vi "XY Graph TipStrip Mouse Move.vi"(4 "Top/Bottom(F)":bool, 5 "Max Length (200)":i32=200, 6 "Left/Right(F)":bool, 7 "Offset (10)":i32=10, 8 "Error In":errorcluster, 10 "Coords":T1, 11 "XY Graph Refnum":T2) -> (0 "Error Out":errorcluster, 1 "Plot Name":string, 2 "Plot at Coordinates":i32)   [LabVIEW 2019, in "XY Graph Add-Ons.lvlib"]
doc: "Shows a tipstrip indicating the name of the plot in the graph legend over which the mouse is located.\n\nThe maximal length (<b>Max Length</b>)of the tipstrip is optional (default: 200 pixels).\nThe relative location of the tipstrip (with respect to the mouse) can be specified with two flags (<b>Top/Bottom</b> and <b>Left/Right</b>) and an <b>Offset</b> value.\nThe default is bottom right, with an offset of 10 pixels in both directions.\n\nIf the mouse is over a plot legend, its index and legend are returned. Otherwise -1 and an empty string are returned."
uses:
  XY Graph Add-Ons.lvlib
  XY Graph Refnum.ctl
  <vilib>/Utility/miscctls.llb/LVPoint32TypeDef.ctl
  <vilib>/Utility/miscctls.llb/LVPositionTypeDef.ctl
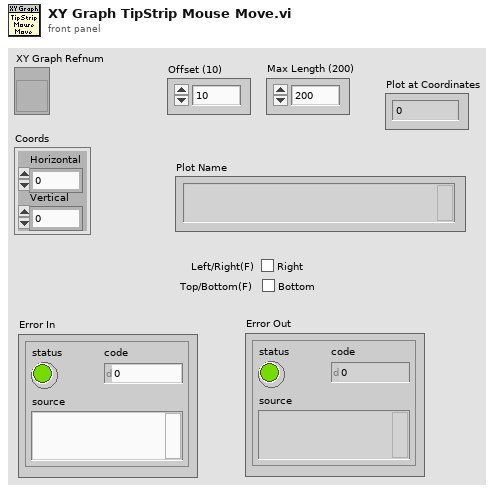
[diagram p1: front panel]
types:
  T1 = typedef "LVPoint32TypeDef.ctl" = cluster{"Horizontal":i32, "Vertical":i32}
  T2 = typedef "XY Graph Add-Ons.lvlib/XY Graph Refnum.ctl" = refnum<vi>
  T3 = typedef "LVPositionTypeDef.ctl" = cluster{"Left":i32, "Top":i32}
  T4 = typedef "LVPointTypeDef.ctl" = cluster{"Horizontal":i16, "Vertical":i16}
  T5 = typedef "LVBoundsTypeDef.ctl" = cluster{"Width":u32, "Height":u32}
  T6 = cluster{"left":i16, "top":i16, "right":i16, "bottom":i16}
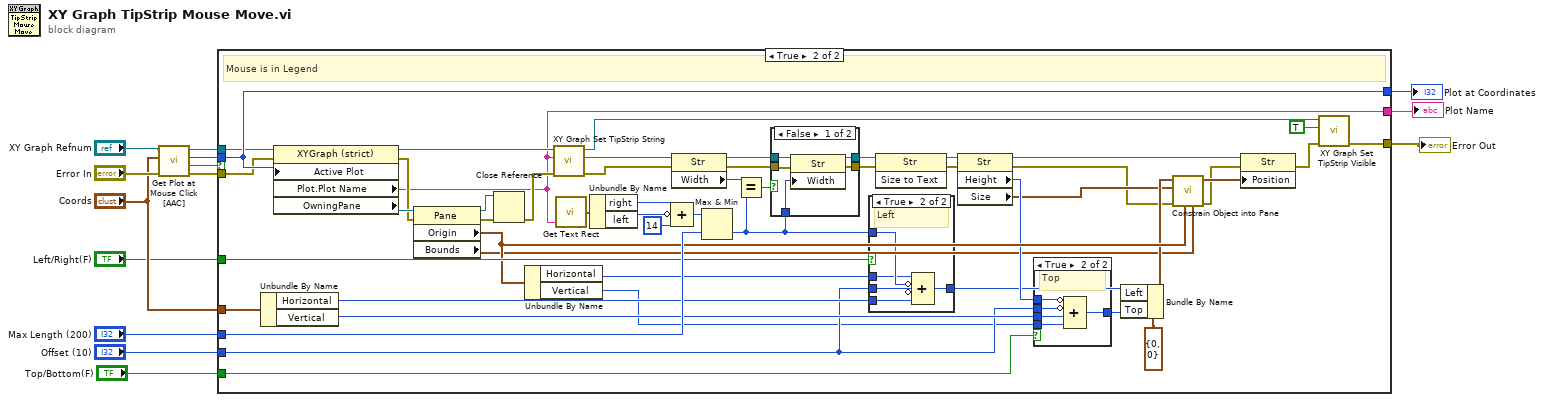
[diagram p0: block diagram]
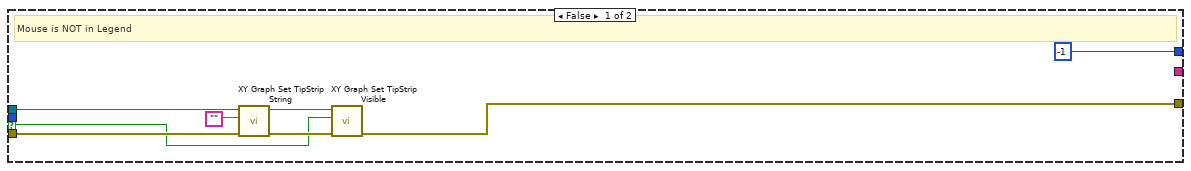
[diagram p2: hidden frame]
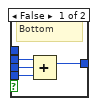
[diagram p3: hidden frame]
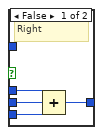
[diagram p4: hidden frame]
diagram:
  n1 = call "Get Plot at Mouse Click [AAC].vi"("error in (no error)"="Error In", "Mouse Click Coordinates"="Coords", "XYGraph Ref"="XY Graph Refnum") -> ("error out"=w1:errorcluster, "Click is in Legend?"=w12:bool, "Plot at Coordinates"=w11:i32, "XYGraph Ref"=w2:T2)  [unwired: 2 in, 3 out]
  n2 = case shown="True" w12 {
    selector: w12 -> [w18 _]
    tunnel: w11 -> [_ w63]
    tunnel: [w16 w26] -> w10
    tunnel: "Coords" -> [_ w71]
    tunnel: [_ w24] -> w8
    tunnel: "Max Length (200)" -> [_ w73]
    tunnel: "Left/Right(F)" -> [_ w72]
    tunnel: "Top/Bottom(F)" -> [_ w70]
    tunnel: "Offset (10)" -> [_ w67]
    tunnel: [-1 ("Plot at Coordinates") w63] -> w3
    tunnel: w2 -> [w17 w60]
    tunnel: w1 -> [w20 w33]
    frame False {
      # "Mouse is NOT in Legend"
      n3 = call "XY Graph Set TipStrip String.vi"("error in (no error)"=w20, "TipStrip String"="", "XY Graph Refnum"=w17) -> ("error out"=w19:errorcluster, "XY Graph Refnum (dup)"=w15:T2)  [unwired: 6 in, 1 out]
      n4 = call "XY Graph Set TipStrip Visible.vi"("error in (no error)"=w19, "TipStrip Visible"=w18, "XY Graph Refnum"=w15) -> ("error out"=w16:errorcluster)  [unwired: 6 in, 2 out]
    }
    frame True {
      # "Mouse is in Legend"
      n5 = Unbundle By Name(w71) -> ("Horizontal"=w68:i32, "Vertical"=w69:i32)
      n6 = property class="XYGraph (strict)"(reference=w60, error in=w33, "Active Plot"=w63) -> (reference out=w32:T2, error out=w65:errorcluster, "Plot.Plot Name"=w24:string, "OwningPane"=w66:refnum<vi>)
      n7 = property class="Pane"(reference=w66, error in=w65) -> (reference out=w62:refnum<vi>, error out=w61:errorcluster, "Origin"=w64:T4, "Bounds"=w23:T5)
      n8 = Close Reference(reference=w62, error in (no error)=w61) -> (error out=w29:errorcluster)
      n9 = Unbundle By Name(w64) -> ("Horizontal"=w37:i16, "Vertical"=w36:i16)
      n10 = call "XY Graph Set TipStrip String.vi"("error in (no error)"=w29, "TipStrip String"=w24, "XY Graph Refnum"=w32) -> ("error out"=w30:errorcluster, "TipStrip Refnum"=w31:refnum<vi>, "XY Graph Refnum (dup)"=w28:T2)  [unwired: 6 in]
      n11 = call <vilib>:"Get Text Rect.vi"("text"=w24) -> ("rect"=w59:T6)  [unwired: 8 in]
      n12 = Unbundle By Name(w59) -> ("right"=w58:i16, "left"=w57:i16)
      n13 = Compound Arithmetic op=ADD(w58, invert w57, i16 14 ("value")) -> (w55:i16)
      n14 = property class="Str"(reference=w31, error in=w30) -> (reference out=w52:refnum<vi>, error out=w51:errorcluster, "Width"=w54:u32)
      n15 = Max & Min(x=w55, y=w73) -> (min(x,y)=w45:i32)  [unwired: 1 out]
      n16 = Equal?(x=w54, y=w45) -> (x = y?=w53:bool)
      n17 = case shown="False" w53 {
        tunnel: w52 -> [w96 w98]
        tunnel: w51 -> [w95 w97]
        tunnel: [w94 w98] -> w50
        tunnel: [w93 w97] -> w49
        tunnel: w45 -> [w92 _]
        frame False {
          n18 = property class="Str"(reference=w96, error in=w95, "Width"=w92) -> (reference out=w94:refnum<vi>, error out=w93:errorcluster)
        }
        frame True {
        }
      }
      n19 = case shown="True" w72 {
        tunnel: w45 -> [_ w89]
        tunnel: w68 -> [w86 w91]
        tunnel: w67 -> [w85 w90]
        tunnel: [w84 w88] -> w41
        tunnel: w37 -> [w83 w87]
        frame False {
          # "Right"
          n20 = Compound Arithmetic op=ADD(w83, w85, w86) -> (w84:i32)
        }
        frame True {
          # "Left"
          n21 = Compound Arithmetic op=ADD(w87, invert w89, invert w90, w91) -> (w88:i32)
        }
      }
      n22 = invoke class="Str" method="Size to Text"(reference=w50, error in=w49) -> (reference out=w48:refnum<vi>, error out=w47:errorcluster)  [unwired: 1 in, 1 out]
      n23 = property class="Str"(reference=w48, error in=w47) -> (reference out=w46:refnum<vi>, error out=w35:errorcluster, "Height"=w42:u32, "Size"=w38:T5)
      n24 = case shown="True" w70 {
        tunnel: w69 -> [w77 w82]
        tunnel: w67 -> [w76 w81]
        tunnel: [w75 w80] -> w43
        tunnel: w42 -> [_ w79]
        tunnel: w36 -> [w74 w78]
        frame False {
          # "Bottom"
          n25 = Compound Arithmetic op=ADD(w76, w77, w74) -> (w75:i32)
        }
        frame True {
          # "Top"
          n26 = Compound Arithmetic op=ADD(invert w79, invert w81, w82, w78) -> (w80:u32)
        }
      }
      n27 = Bundle By Name(cluster=T3 {"Left"=0, "Top"=0} ("Position"), "Left"=w41, "Top"=w43) -> (w39:T3)
      n28 = call "Constrain Object into Pane.vi"("Pane Bounds"=w23, "Panel Origin"=w64, "Error In"=w35, "Object Size"=w38, "Object Position in"=w39) -> ("Error Out"=w34:errorcluster, "Object Position out"=w40:T3)  [unwired: 5 in]
      n29 = property class="Str"(reference=w46, error in=w34, "Position"=w40) -> (error out=w27:errorcluster)  [unwired: 1 out]
      n30 = call "XY Graph Set TipStrip Visible.vi"("error in (no error)"=w27, "TipStrip Visible"=TRUE, "XY Graph Refnum"=w28) -> ("error out"=w26:errorcluster)  [unwired: 6 in, 2 out]
    }
  }
  "Error Out" <- w10
  "Plot Name" <- w8
  "Plot at Coordinates" <- w3
